vi "GA Get Ctrl Mode.vi"(8 "error in (no error)":errorcluster caption="错误输入（无错误）", 10 "pMode":i16, 11 "nAxisNum":i16) -> (0 "error out":errorcluster caption="错误输出", 2 "pMode out":i16, 3 "function return":i32)   [LabVIEW 2015, in "GAS.lvlib"]
doc: "extern \"C\" __declspec(dllimport) int GA_GetCtrlMode(short nAxisNum,short *pMode);"
uses:
  <userlib>/BP_GAS/GAS.lvlib
  <userlib>/BP_GAS/GAS.dll
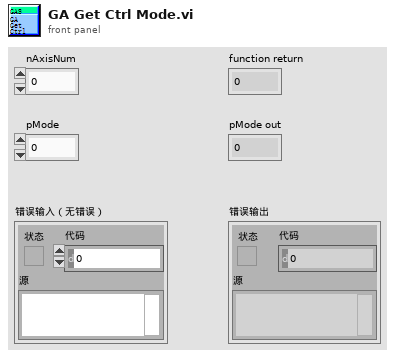
[diagram p1: front panel]
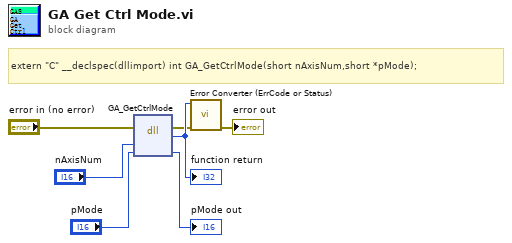
[diagram p0: block diagram]
diagram:
  # "extern \"C\" __declspec(dllimport) int GA_GetCtrlMode(short nAxisNum,short *pMode);"
  n1 = dll-call lib="E:/Program Files (x86)/National Instruments/LabVIEW 2015/user.lib/BP_GAS/GAS.*" fn="GA_GetCtrlMode"(error in="error in (no error)", "nAxisNum"="nAxisNum", "pMode"="pMode") -> (error out=w2:errorcluster, w7:i32, "pMode"=→"pMode out":i16)  [unwired: 3 in, 1 out]
  "function return" <- w7
  n2 = call "Error Converter (ErrCode or Status).vi"("error in (no error)"=w2, "error code"=w7) -> ("error out"=→"error out":errorcluster)  [unwired: 9 in]
